vi "Configure Sweep Mode.vi"(8 "error in (no error)":errorcluster, 10 "Sweep Mode":enum16{"Continuous", "Single"}(ring), 11 "Spectrum Analyzer in":refnum<class "Spectrum Analyzer.lvclass">) -> (0 "error out":errorcluster, 3 "Spectrum Analyzer out":refnum<class "Spectrum Analyzer.lvclass">)   [LabVIEW 2020, in "Spectrum Analyzer.lvclass"]
uses:
  Spectrum Analyzer.lvclass
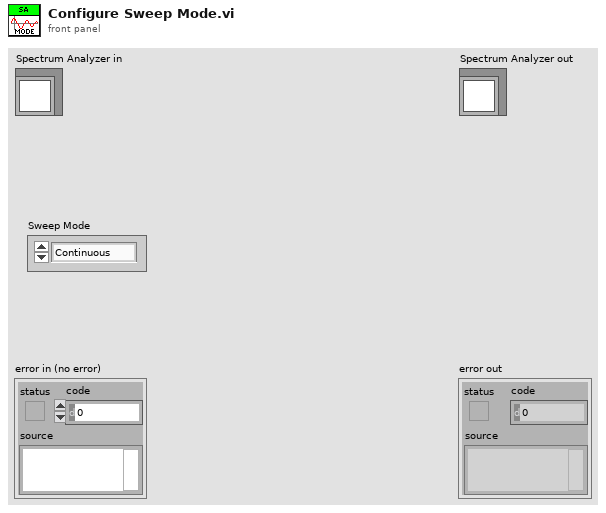
[diagram p1: front panel]
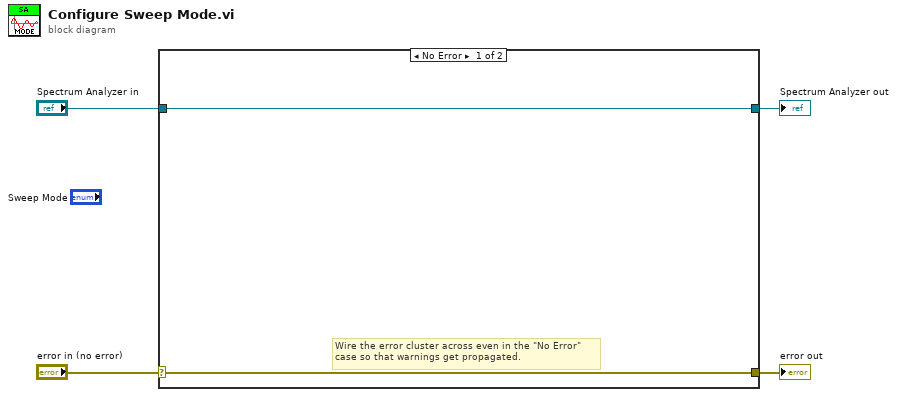
[diagram p0: block diagram]
diagram:
  n1 = case shown="No Error" "error in (no error)" {
    selector: "error in (no error)" -> [w5 w8]
    tunnel: [w5 w8] -> w3
    tunnel: [w6 w7] -> w1
    tunnel: "Spectrum Analyzer in" -> [w6 w7]
    frame No Error {
      # "Wire the error cluster across even in the \"No Error\"\ncase so that warnings get propagated."
    }
    frame Error {
    }
  }
  "error out" <- w3
  "Spectrum Analyzer out" <- w1
